vi "WebPowerSwitchOff.vi"() -> (5 "Plug in titles":string[](array[string]), 7 "Plug in values":string[](array[string]))   [LabVIEW 2020]
uses:
  ADAM Client/Sub VIs/ADAM Controls/Ch_description_ADAM.ctl
  ADAM Client/Sub VIs/ADAM Controls/Module_type_ADAM.ctl
  ADAM Client/Sub VIs/ADAM Controls/Function_ADAM.ctl
  ADAM Client/Sub VIs/ADAM Controls/Channel_State.ctl
  ADAM Client/Sub VIs/ADAM Controls/Calib_type_ADAM.ctl
  ADAM Client/Sub VIs/ADAM Controls/Address.ctl
  Globals/Meas_global.vi
panel:
  in  "WebPowerSwitchIP":string="10.245.69.7"
  in  "WebPowerSwitchOutlet":i32=1
  in  "DesiredState":bool
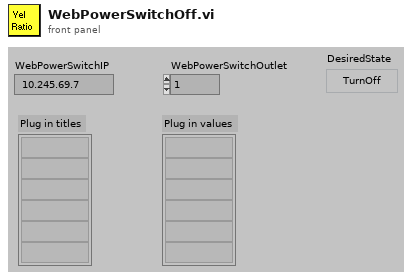
[diagram p1: front panel]
types:
  T1 = typedef "Post_Process.ctl" = enum16{"Take New Data", "Post Process Raw Data File"}
  T2 = typedef "Ch_description_ADAM.ctl" = cluster{"Ch Name":string, "Type":T3, "Function":T4, "Ch State":T5, "Calibration type":T6, "A":dbl, "B":dbl, "C":dbl, "D":dbl, "Comments":string, "Address":T7, "String":string, "Duty":u16}
  T3 = typedef "Module_type_ADAM.ctl" = string
  T4 = typedef "Function_ADAM.ctl" = enum16{"Analogue Input", "Digital Input", "Event counter", "Event rate", "Analogue Output", "Digital Output", "Relay Output"}
  T5 = typedef "Channel_State.ctl" = enum16{"On", "Off", "Always On", "Always Off"}
  T6 = typedef "Calib_type_ADAM.ctl" = string
  T7 = typedef "Address.ctl" = cluster{"Main":i32, "Ch.":i32, "Sub":i32, "Port Name":string}
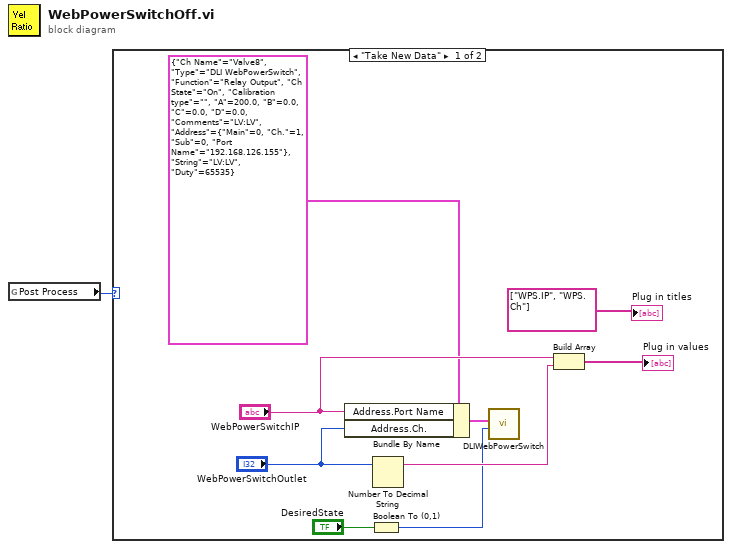
[diagram p0: block diagram]
diagram:
  n1 = global read "Meas_global.vi" "Post Process"() -> (w1:T1)
  n2 = case shown="\"Take New Data\"" w1 {
    frame "Take New Data" {
      n3 = Bundle By Name(cluster=T2 {"Ch Name"="Valve8", "Type"="DLI WebPowerSwitch", "Function"=enum."Relay Output", "Ch State"=enum."On", "Calibration type"="", "A"=200.0, "B"=0.0, "C"=0.0, "D"=0.0, "Comments"="LV:LV", "Address"={"Main"=0, "Ch."=1, "Sub"=0, "Port Name"="192.168.126.155"}, "String"="LV:LV", "Duty"=65535} ("Ch Description"), "Address.Port Name"="WebPowerSwitchIP", "Address.Ch."="WebPowerSwitchOutlet") -> (w4:T2)
      n4 = Boolean To (0,1)(Boolean="DesiredState") -> (0, 1=w7:i16)
      n5 = Number To Decimal String(number="WebPowerSwitchOutlet") -> (decimal integer string=w10:string)  [unwired: 1 in]
      n6 = call "DLIWebPowerSwitch.vi"("Value to Output"=w7, "Ch Description"=w4) -> ()  [unwired: 5 in, 3 out]
      n7 = Build Array("WebPowerSwitchIP", w10) -> (→"Plug in values":string[])
      "Plug in titles" <- string[] ["WPS.IP", "WPS.Ch"] ("Plug in titles")
    }
    frame "Post Process Raw Data File" {
    }
  }
